vi "asset.get_from_datasouce.request.vi"(8 "error in":errorcluster) -> (0 "error out":errorcluster, 3 "request":string)   [LabVIEW 2020, in "Nominal Client.lvclass"]
uses:
  Nominal Client.lvclass
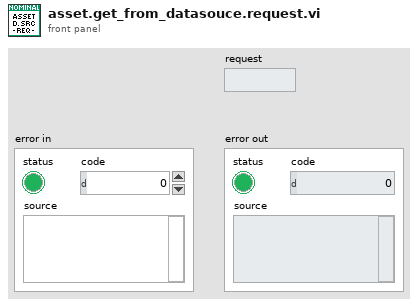
[diagram p1: front panel]
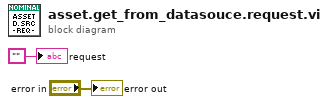
[diagram p0: block diagram]
diagram:
  "error out" <- "error in"
  "request" <- ""
